vi "RDB Receive.vi"(8 "error in (no error)":errorcluster, 10 "RDB Reference in":T4 {"RDB Send Reference"."RDB Data"."payload" format="%x"; "RDB Send Reference"."RDB Data"."timestamp" format="%<%.7X\n%x>T"; "RDB Send Reference"."RDB Data"."type" items=["FlexRay Data"=32, "FlexRay Null"=33, "FlexRay Symbol"=34, "Log Trigger"=225, "Start Trigger"=226]; "RDB Send Reference"."RDB Data"."cycle count" max=63 step=1; "RDB Receive Reference"."RDB Data"."payload" format="%x"; "RDB Receive Reference"."RDB Data"."timestamp" format="%<%.7X\n%x>T"; "RDB Receive Reference"."RDB Data"."type" items=["FlexRay Data"=32, "FlexRay Null"=33, "FlexRay Symbol"=34, "Log Trigger"=225, "Start Trigger"=226]; "RDB Receive Reference"."RDB Data"."cycle count" max=63 step=1}, 11 "Settings":T1={"UDP Receiver"=refnum, "UDP Sender"=refnum, "Valid Packet"=FALSE, "TCP"=refnum, "Network Settings"={"IP adress"="127.0.0.1", "RDB"={"Protocol"=enum."UDP", "Tx Port"=48270, "Rx Port"=10, "Buffer Size"=204800, "Timeout"=10}, "SCP"={"Protocol"=enum."TCP", "Tx Port"=48191, "Rx Port"=48191, "Buffer Size"=204800, "Timeout"=10}}, "vclient"=path ""}) -> (0 "error out":errorcluster, 2 "RDB Reference out":T4 {"RDB Send Reference"."RDB Data"."payload" format="%x"; "RDB Send Reference"."RDB Data"."timestamp" format="%<%.7X\n%x>T"; "RDB Send Reference"."RDB Data"."type" items=["FlexRay Data"=32, "FlexRay Null"=33, "FlexRay Symbol"=34, "Log Trigger"=225, "Start Trigger"=226]; "RDB Send Reference"."RDB Data"."cycle count" max=63 step=1; "RDB Receive Reference"."RDB Data"."payload" format="%x"; "RDB Receive Reference"."RDB Data"."timestamp" format="%<%.7X\n%x>T"; "RDB Receive Reference"."RDB Data"."type" items=["FlexRay Data"=32, "FlexRay Null"=33, "FlexRay Symbol"=34, "Log Trigger"=225, "Start Trigger"=226]; "RDB Receive Reference"."RDB Data"."cycle count" max=63 step=1}, 3 "Settings":T1={"UDP Receiver"=refnum, "UDP Sender"=refnum, "Valid Packet"=FALSE, "TCP"=refnum, "Network Settings"={"IP adress"="127.0.0.1", "RDB"={"Protocol"=enum."UDP", "Tx Port"=48270, "Rx Port"=10, "Buffer Size"=204800, "Timeout"=10}, "SCP"={"Protocol"=enum."TCP", "Tx Port"=48191, "Rx Port"=48191, "Buffer Size"=204800, "Timeout"=10}}, "vclient"=path ""})   [LabVIEW 2023, in "RDB.lvlib"]
uses:
  RDB.lvlib
  RDB References.ctl
  RDB Reference.ctl
  <vilib>/xnet/xnet.llb/XNET Frame FlexRay.ctl
  <vilib>/xnet/xnet.llb/XNET Frame Type FlexRay.ctl
  Engine/Type/Settings.ctl
  Shared/Network Settings.ctl
  Shared/Protocol.ctl
  <vilib>/xnet/xnet.llb/XNET Convert (Frame FlexRay to Signal).vi
  Engine/Vires VTD Engine.lvlib
  Shared/Vires VTD Shared.lvlib
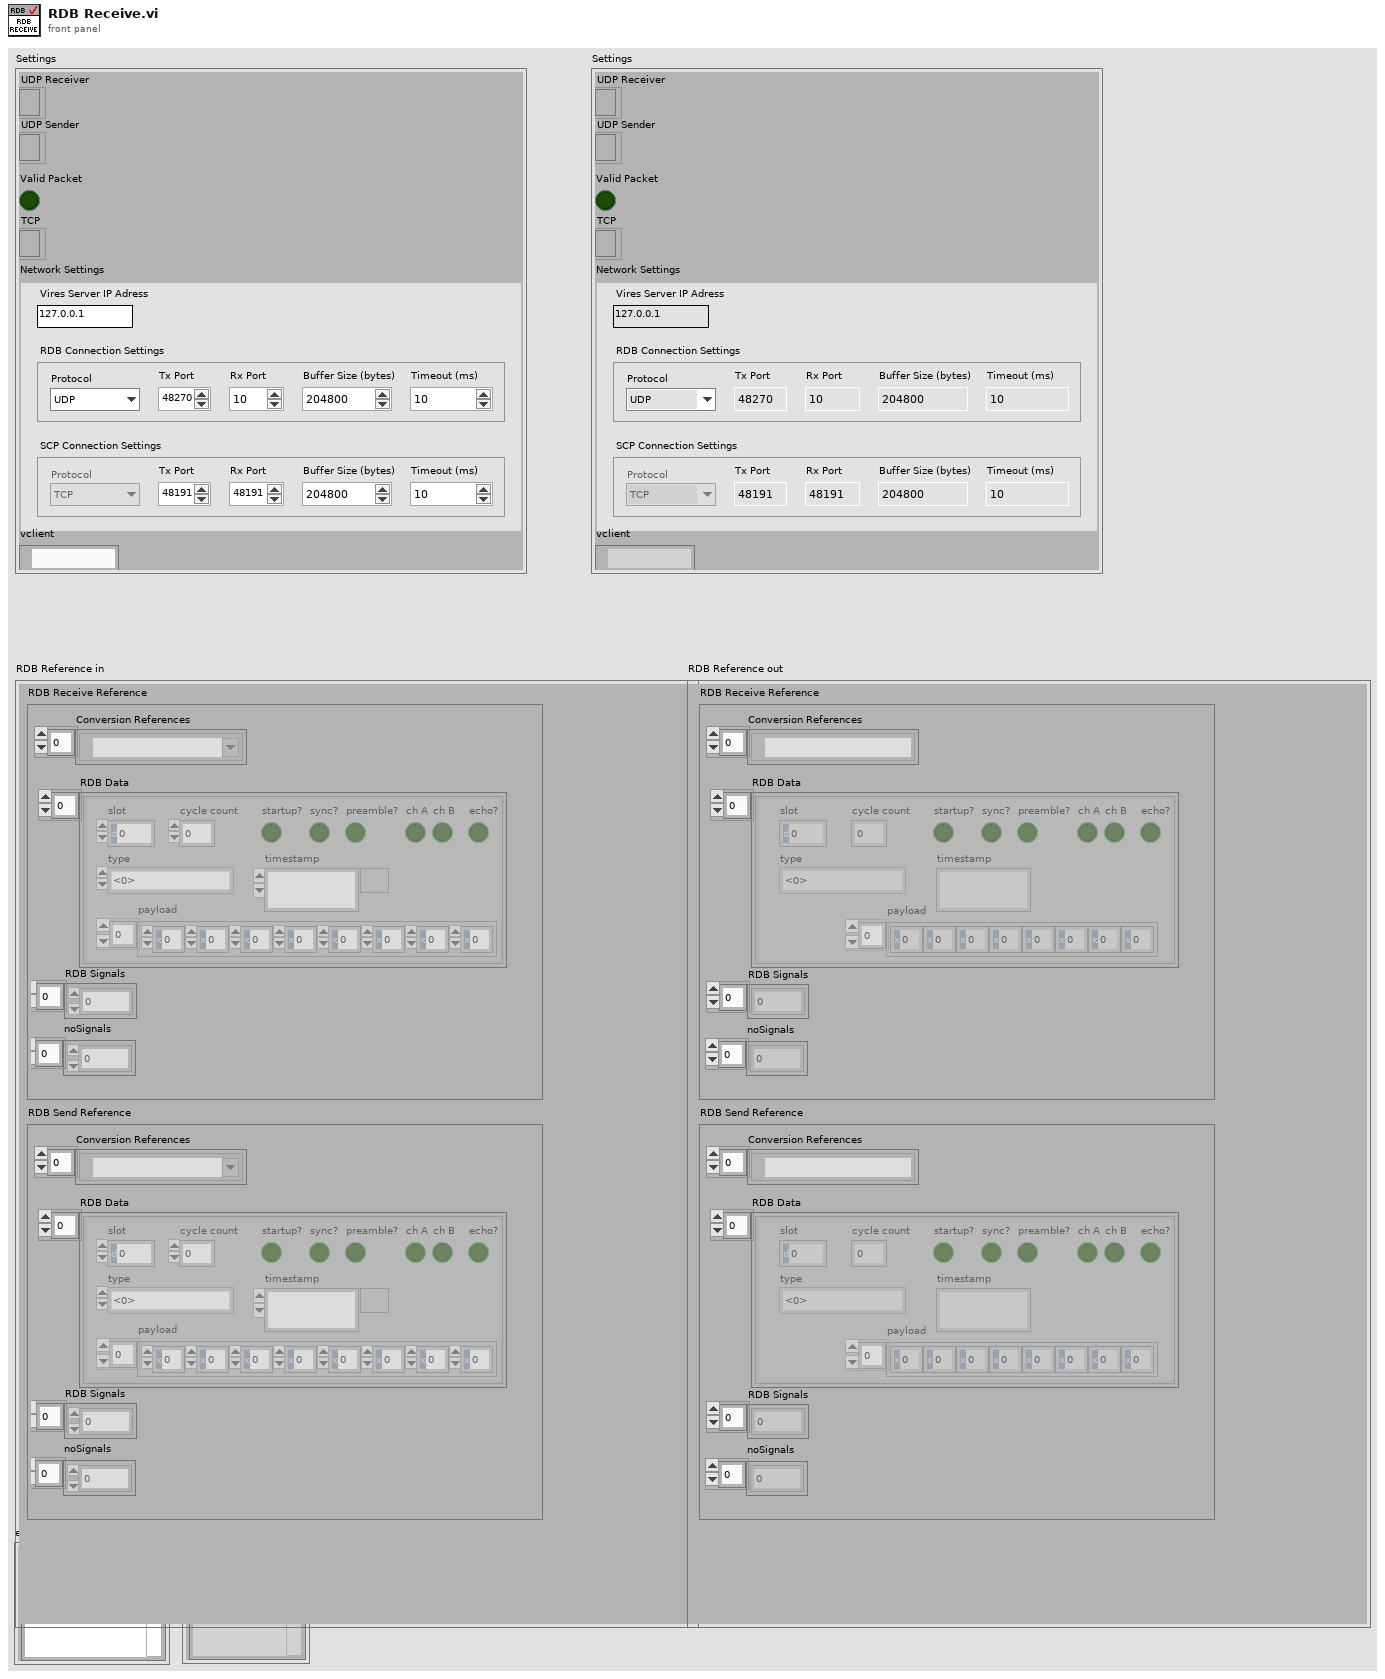
[diagram p1: front panel]
types:
  T1 = typedef "Vires VTD Engine.lvlib/Settings.ctl" = cluster{"UDP Receiver":refnum<k16>, "UDP Sender":refnum<k16>, "Valid Packet":bool, "TCP":refnum<k5>, "Network Settings":T2, "vclient":path}
  T2 = typedef "Vires VTD Shared.lvlib/Network Settings.ctl" = cluster{"IP adress":string, "RDB":cluster{"Protocol":T3, "Tx Port":u16, "Rx Port":u16, "Buffer Size":i32, "Timeout":u16}, "SCP":cluster{"Protocol":T3, "Tx Port":u16, "Rx Port":u16, "Buffer Size":i32, "Timeout":u16}}
  T3 = typedef "Vires VTD Shared.lvlib/Protocol.ctl" = enum16{"UDP", "TCP"}
  T4 = typedef "RDB.lvlib/RDB References.ctl" = cluster{"RDB Receive Reference":T5, "RDB Send Reference":T5}
  T5 = typedef "RDB.lvlib/RDB Reference.ctl" = cluster{"Conversion References":refnum<k21>[], "RDB Data":T6[], "RDB Signals":dbl[], "noSignals":i32[]}
  T6 = typedef "XNET Frame FlexRay.ctl" = cluster{"timestamp":timestamp, "payload":u8[], "slot":u16, "type":T7, "cycle count":u8, "startup?":bool, "sync?":bool, "preamble?":bool, "ch A":bool, "ch B":bool, "echo?":bool}
  T7 = typedef "XNET Frame Type FlexRay.ctl" = u8
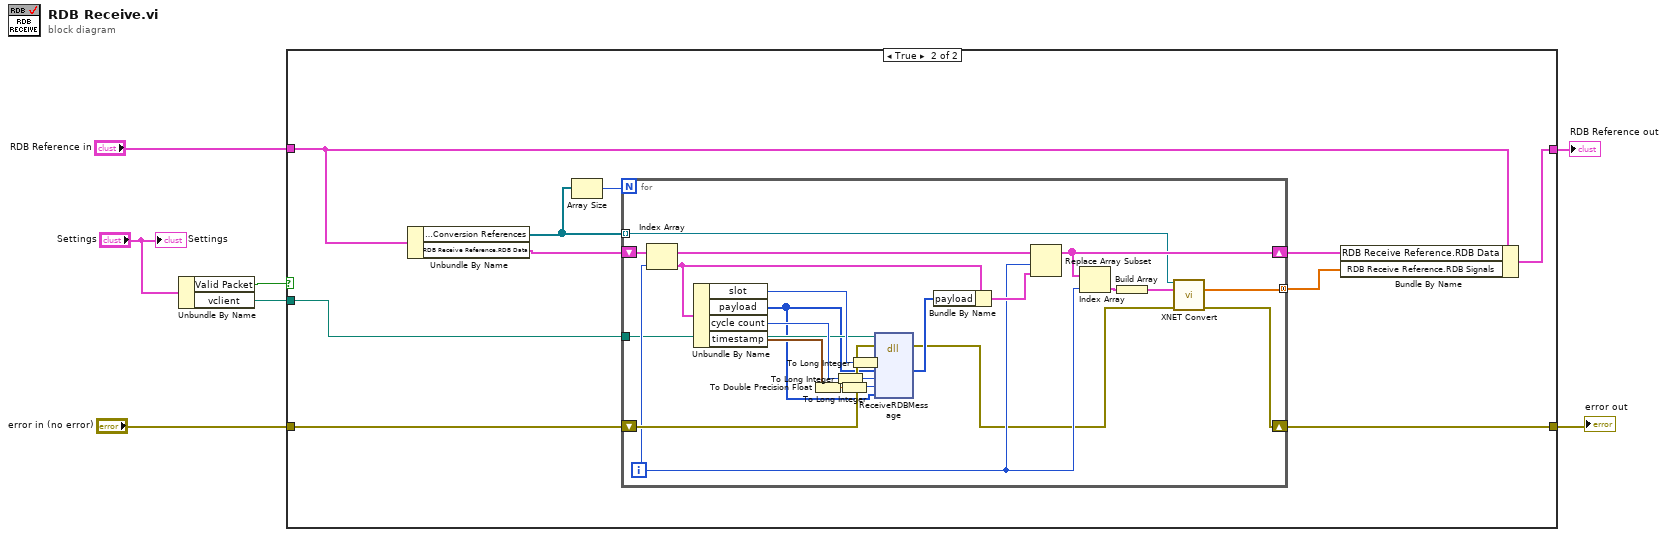
[diagram p0: block diagram]
diagram:
  n1 = Unbundle By Name("Settings") -> ("Valid Packet"=w3:bool, "vclient"=w1:path)
  n2 = case shown="True" w3 {
    tunnel: "RDB Reference in" -> [w9 w19]
    tunnel: [w9 w18] -> w6
    tunnel: "error in (no error)" -> [w8 w12]
    tunnel: [w8 w11] -> w4
    tunnel: w1 -> [_ w10]
    frame False {
    }
    frame True {
      n3 = Unbundle By Name(w19) -> ("RDB Receive Reference.Conversion References"=w14:refnum<k21>[], "RDB Receive Reference.RDB Data"=w16:T6[])
      n4 = Array Size(array=w14) -> (size(s)=w15:i32)
      n5 = for {
        N: w15 -> [_]
        shift-right: [w28] -> w11
        shift-left: w12 -> [w39]
        tunnel: w14 -> [w31] mode=indexing
        shift-right: [w34] -> w17
        shift-left: w16 -> [w36]
        tunnel: [w27] -> w13 mode=concatenating
        tunnel: w10 -> [w26]
        i -> [w33]
        n6 = Index Array(array=w36, index=w33) -> (element=w37:T6)
        n7 = Unbundle By Name(w37) -> ("slot"=w41:u16, "payload"=w20:u8[], "cycle count"=w38:u8, "timestamp"=w24:timestamp)
        n8 = To Double Precision Float(number=w24) -> (double precision float=w25:dbl)
        n9 = To Long Integer(number=w38) -> (32bit integer=w23:i32)
        n10 = To Long Integer(number=w25) -> (32bit integer=w21:i32)
        n11 = To Long Integer(number=w41) -> (32bit integer=w22:i32)
        n12 = dll-call lib="E:/Documents/Systems Engineering/Custom VeriStand Development/Vires VTD Custom Device/Vires VTD Custom Device/Vires VTD/Source/RDB/vclient.*" fn="ReceiveRDBMessage"(path in=w26, error in=w39, "ID"=w22, "Item"=w20, "id"=w23, "wheelid"=w21, "Data"=w20) -> (error out=w29:errorcluster, "Item"=w40:u8[])  [unwired: 6 in, 1 out]
        n13 = Bundle By Name(cluster=w37, "payload"=w40) -> (w35:T6)
        n14 = Replace Array Subset(array=w36, new element=w35, index=w33) -> (w34:T6[])
        n15 = Index Array(array=w34, index=w33) -> (element=w32:T6)
        n16 = Build Array(w32) -> (w30:T6[])
        n17 = call-poly <vilib>:"XNET Convert.vi"("session in"=w31, "frame data"=w30, "error in (no error)"=w29) -> ("signal data"=w27:dbl[], "error out"=w28:errorcluster)  [unwired: 10 in, 1 out]
      }
      n18 = Bundle By Name(cluster=w19, "RDB Receive Reference.RDB Data"=w17, "RDB Receive Reference.RDB Signals"=w13) -> (w18:T4)
    }
  }
  "RDB Reference out" <- w6
  "error out" <- w4
  "Settings" <- "Settings"
